vi "Extract_cluster_from_XML.vi"(0 "XML_Cluster_String":string) -> (1 "Cluster":string, 2 "AfterCluster":string)   [LabVIEW 2011]
panel:
  out "nesting_level":i32
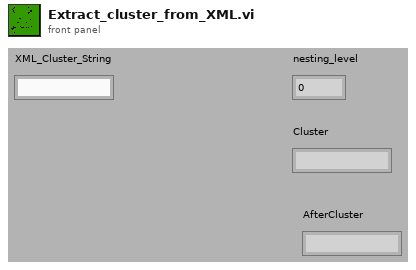
[diagram p1: front panel]
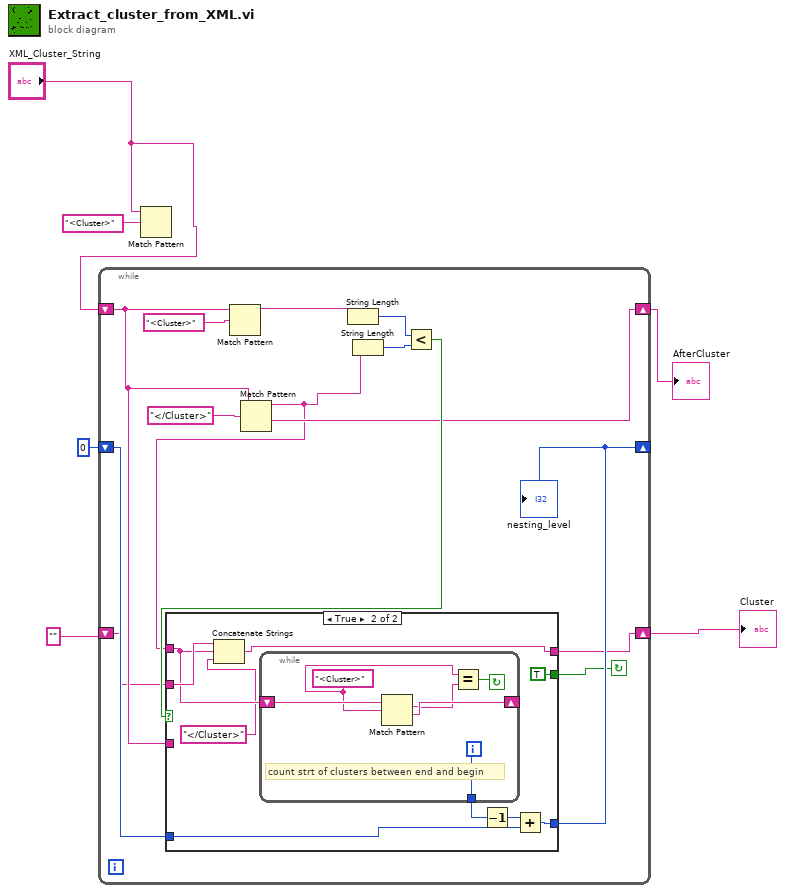
[diagram p0: block diagram]
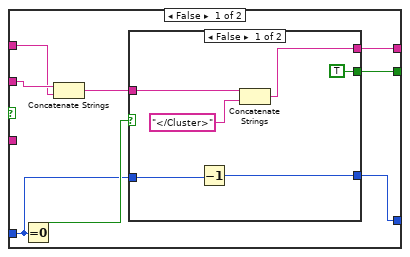
[diagram p2: hidden frame]
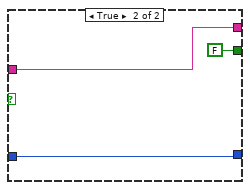
[diagram p3: hidden frame]
diagram:
  n1 = while {
    shift-right: [w11] -> w2
    shift-left: "XML_Cluster_String" -> [w10]
    shift-right: [w13] -> _
    shift-left: 0 -> [w14]
    shift-right: [w7] -> w6
    shift-left: "" ("after substring") -> [w8]
    stop <- w12 continue-if-true
    n2 = Match Pattern(string=w10, regular expression="<Cluster>") -> (before substring=w18:string)  [unwired: 1 in, 3 out]
    n3 = Match Pattern(string=w10, regular expression="</Cluster>") -> (before substring=w9:string, after substring=w11:string)  [unwired: 1 in, 2 out]
    n4 = String Length(string=w18) -> (length=w17:i32)
    n5 = String Length(string=w9) -> (length=w16:i32)
    n6 = Less?(x=w17, y=w16) -> (x < y?=w15:bool)
    n7 = case shown="True" w15 {
      tunnel: w9 -> [w25 w42]
      tunnel: w14 -> [w22 w46]
      tunnel: [w21 w45] -> w13
      tunnel: [w27 TRUE] -> w12
      tunnel: w10 -> [_ _]
      tunnel: w8 -> [w26 w43]
      tunnel: [w23 w40] -> w7
      frame False {
        n8 = Equal To 0?(x=w22) -> (x = 0?=w28:bool)
        n9 = Concatenate Strings(w26, w25) -> (w24:string)
        n10 = case shown="False" w28 {
          tunnel: [TRUE FALSE] -> w27
          tunnel: w24 -> [w34 w36]
          tunnel: [w32 w36] -> w23
          tunnel: w22 -> [w31 w35]
          tunnel: [w30 w35] -> w21
          frame False {
            n11 = Decrement(x=w31) -> (x-1=w30:i32)
            n12 = Concatenate Strings(w34, "</Cluster>" ("regular expression")) -> (w32:string)
          }
          frame True {
          }
        }
      }
      frame True {
        n13 = Concatenate Strings(w43, w42, "</Cluster>" ("regular expression")) -> (w40:string)
        n14 = while {
          shift-right: [w51] -> _
          shift-left: w42 -> [w52]
          tunnel: [w47] -> w39
          i -> [w47]
          stop <- w48 continue-if-true
          w50 = "<Cluster>" ("regular expression")
          # "count strt of clusters between end and begin"
          n15 = Match Pattern(string=w52, regular expression=w50) -> (match substring=w49:string, after substring=w51:string)  [unwired: 1 in, 2 out]
          n16 = Equal?(x=w50, y=w49) -> (x = y?=w48:bool)
        }
        n17 = Decrement(x=w39) -> (x-1=w38:i32)
        n18 = Add(x=w38, y=w46) -> (x+y=w45:i32)
      }
    }
    "nesting_level" <- w13
  }
  "Cluster" <- w6
  "AfterCluster" <- w2
  n19 = Match Pattern(string="XML_Cluster_String", regular expression="<Cluster>") -> ()  [unwired: 1 in, 4 out]
